vi "Configure Power Meter.vi"(0 "SG Path in":refnum<class "SG Abstract Path.lvclass">, 5 "Cal point in":T1, 11 "error in (no error)":errorcluster) -> (4 "SG Path out":refnum<class "SG Abstract Path.lvclass">, 6 "Cal point out":T1, 15 "error out":errorcluster)   [LabVIEW 2023, in "RFFixtureCharact.Public.lvlib" / "SG Abstract Path.lvclass"]
uses:
  SG Abstract Path.lvclass
  Scalar Path/Type Definitions/Cal Point.ctl
  SG Abstract Path.lvclass/SG Abstract Path.ctl
  Instruments/Power Meter/SG Path PM Accessor Base/SG Path PM Accessor Base.lvclass
  Scalar Path/Scalar Path.lvclass
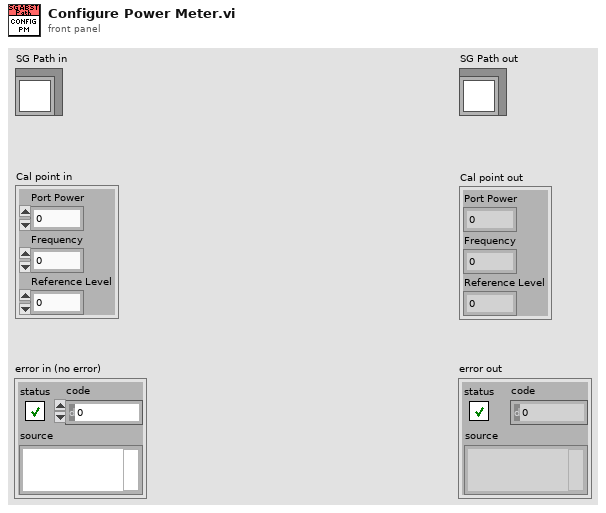
[diagram p1: front panel]
types:
  T1 = typedef "RFFixtureCharact.Public.lvlib/Scalar Path.lvclass/Cal Point.ctl" = cluster{"Port Power":dbl, "Frequency":dbl, "Reference Level":dbl}
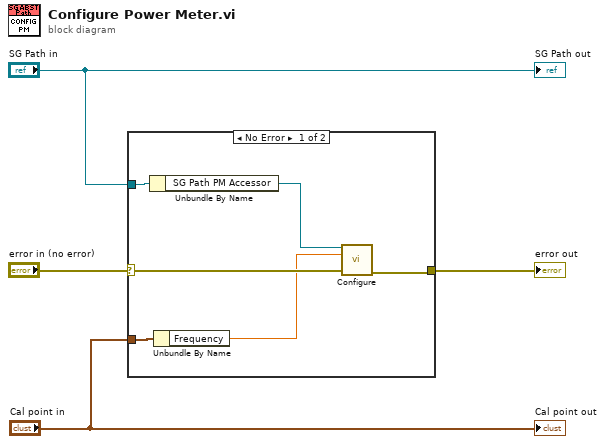
[diagram p0: block diagram]
diagram:
  n1 = case shown="No Error" "error in (no error)" {
    selector: "error in (no error)" -> [w9 w11]
    tunnel: [w8 w11] -> w3
    tunnel: "SG Path in" -> [w10 _]
    tunnel: "Cal point in" -> [w7 _]
    frame No Error {
      n2 = Unbundle By Name(w10) -> ("SG Path PM Accessor"=w6:refnum<class "SG Path PM Accessor Base.lvclass">)
      n3 = Unbundle By Name(w7) -> ("Frequency"=w5:dbl)
      n4 = call-dynamic "Configure.vi"("SG Path Power Meter Accessor in"=w6, "frequency"=w5, "error in (no error)"=w9) -> ("error out"=w8:errorcluster)  [unwired: 11 in, 1 out]
    }
    frame Error {
    }
  }
  "error out" <- w3
  "SG Path out" <- "SG Path in"
  "Cal point out" <- "Cal point in"
